vi "User Dynamic (multiple).vi"(7 "User.Python.lvclass":refnum<class "User.Python.lvclass">, 8 "error in (no error)":errorcluster, 11 "XY-data":cluster{"X-array":dbl[], "Y-array":dbl[]}[](array[cluster]) {"Y-array" format="%.2p"; "X-array" format="%.2p"}) -> (0 "error out":errorcluster, 3 "XY-data out":cluster{"X-array":dbl[], "Y-array":dbl[]}[](array[cluster]) {"Y-array" format="%.2p"; "X-array" format="%.2p"}, 5 "User.Python.lvclass out":refnum<class "User.Python.lvclass">)   [LabVIEW 2019, in "User.Python.lvclass"]
uses:
  User.Python.lvclass
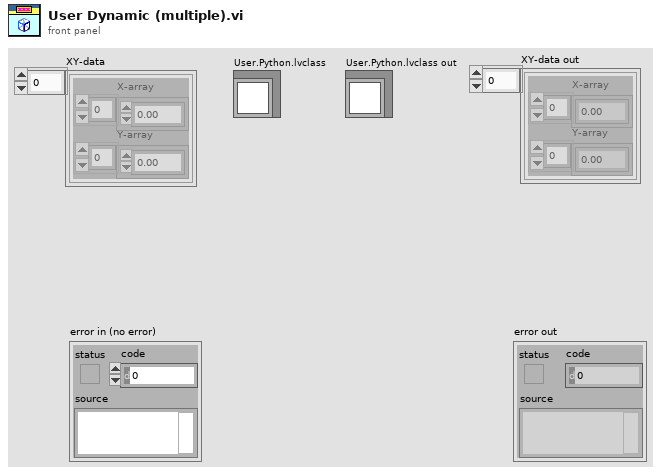
[diagram p1: front panel]
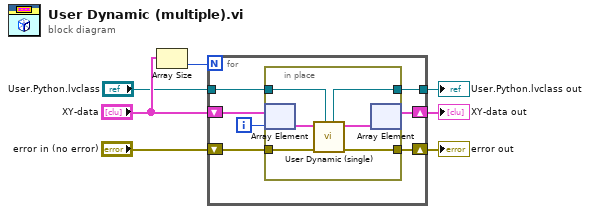
[diagram p0: block diagram]
diagram:
  n1 = Array Size(array="XY-data") -> (size(s)=w7:i32)
  n2 = for {
    N: w7 -> [_]
    tunnel: "User.Python.lvclass" -> [w14]
    shift-right: [w13] -> w3
    shift-left: "XY-data" -> [w9]
    shift-right: [w10] -> w5
    shift-left: "error in (no error)" -> [w11]
    tunnel: [w8] -> w1
    i -> [w12]
    n3 = in-place {
      in-place-border: w14 -> [w16]
      in-place-border: w11 -> [w18]
      in-place-border: [w17] -> w10
      in-place-border: [w15] -> w8
      n4 = in-place-array #1(w9, w12) -> (w20:cluster{"X-array":dbl[], "Y-array":dbl[]})
      n5 = call-dynamic "User Dynamic (single).vi"("User.Python.lvclass"=w16, "error in (no error)"=w18, "XY-data"=w20) -> ("error out"=w17:errorcluster, "XY-data out"=w19:cluster{"X-array":dbl[], "Y-array":dbl[]}, "User.Python.lvclass out"=w15:refnum<class "User.Python.lvclass">)  [unwired: 6 in]
      n6 = in-place-array #1(w19) -> (w13:cluster{"X-array":dbl[], "Y-array":dbl[]}[])  [unwired: 1 out]
    }
  }
  "error out" <- w5
  "XY-data out" <- w3
  "User.Python.lvclass out" <- w1
